vi "libemit.vi"(6 "inparams":string, 8 "error in (no error)":errorcluster, 9 "parameter":string, 10 "function":string, 11 "output":i32) -> (0 "error out":errorcluster)   [LabVIEW 2015]
uses:
  <vilib>/Utility/error.llb/DialogType.ctl
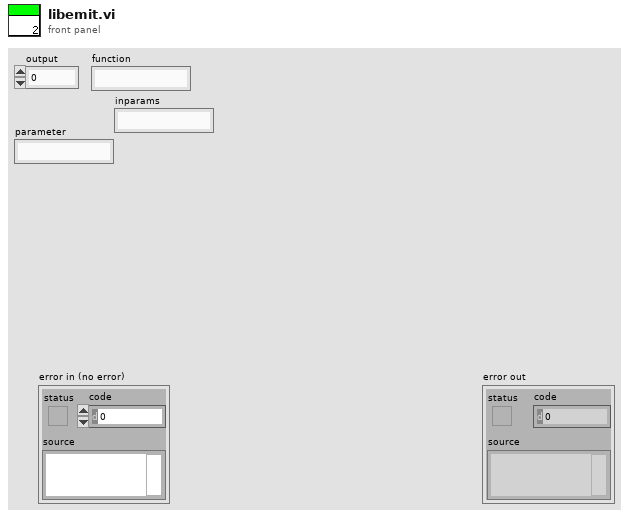
[diagram p1: front panel]
types:
  T1 = typedef "DialogType.ctl" = u16
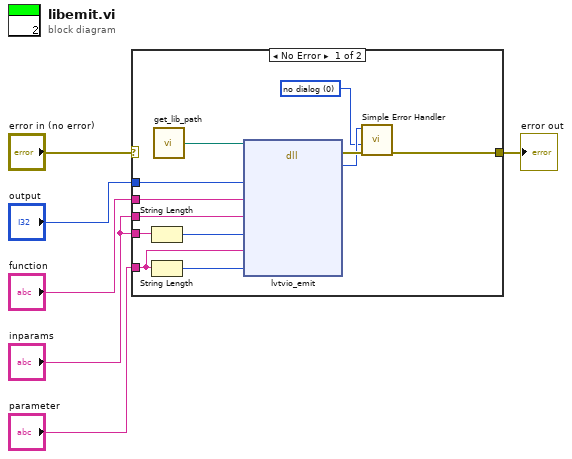
[diagram p0: block diagram]
diagram:
  n1 = case shown="No Error" "error in (no error)" {
    selector: "error in (no error)" -> [_ w19]
    tunnel: [w14 w19] -> w5
    tunnel: "parameter" -> [w13 _]
    tunnel: "function" -> [w12 _]
    tunnel: "inparams" -> [w11 _]
    tunnel: "inparams" -> [w9 _]
    tunnel: "output" -> [w7 _]
    frame No Error {
      w8 = T1 0 items=["no dialog", "OK message", "continue or stop message", "OK message + warnings", "continue/stop + warnings"] ("type of dialog (OK msg:1)")
      n2 = String Length(string=w11) -> (length=w10:i32)
      n3 = String Length(string=w13) -> (length=w15:i32)
      n4 = call "get_lib_path.vi"() -> ("Path"=w18:path)
      n5 = dll-call lib="S:/thingiverselv/lib/liblvtvio.dll" fn="lvtvio_emit"(path in=w18, "output"=w7, "function"=w12, "inparams"=w9, "inparams_size"=w10, "params"=w13, "params_size"=w15) -> (error out=w17:errorcluster, "return type"=w16:i32)  [unwired: 8 in, 1 out]
      n6 = call <vilib>:"Simple Error Handler.vi"("error code (no error:0)"=w16, "type of dialog (OK msg:1)"=w8, "error in (no error)"=w17) -> ("error out"=w14:errorcluster)  [unwired: 2 in, 4 out]
    }
    frame Error {
    }
  }
  "error out" <- w5
